vi "Modify Users.vi"(8 "error In":errorcluster) -> (0 "error Out":errorcluster)   [LabVIEW 2018]
uses:
  Control/Control 7.ctl
panel:
  in  "Login":bool
  in  "New User Type":enum16{"VVDN TECH", "Operator", "QA"}(ring)
  out "Current User Type":enum16{"VVDN TECH", "Operator", "QA"}(ring)
  in  "Stop Button":bool
  in  "Enum":T1
  in  "Selection":string(combo)
  out "Login":bool
  in  "Password":string
  in  "User Name":string(combo)="VVDN TECH"
  in  "Project-Name":string="LensTuning"
  in  "Modify User":bool
  # "MODIFY USERS"
  # "Modify User Details"
  # "Admin Login"
  # "Select User to Modify"
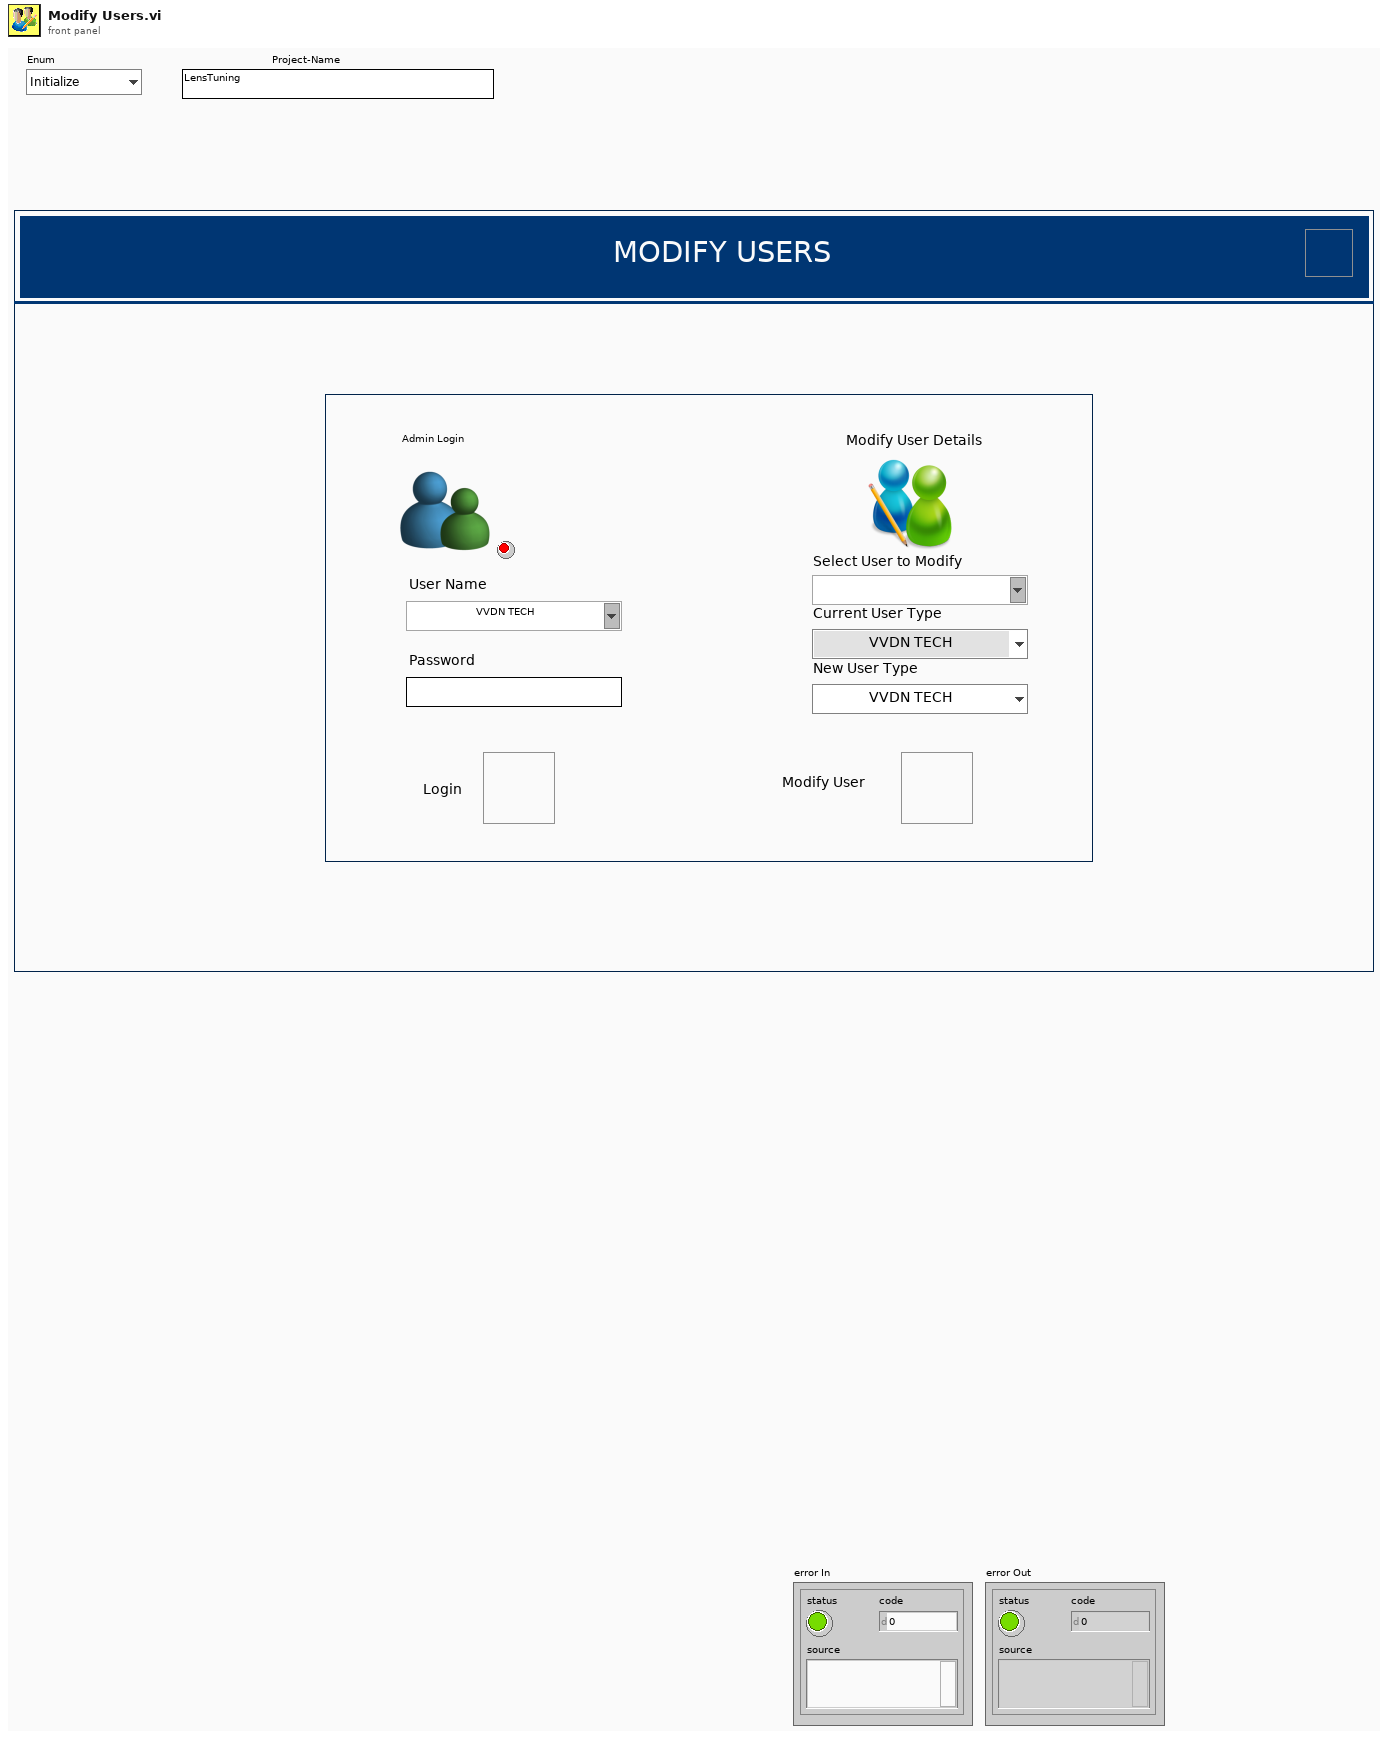
[diagram p1: front panel]
types:
  T1 = typedef "Control 7.ctl" = enum16{"Initialize", "Poll", "Login", "Add User", "Exit"}
  T2 = cluster{"Default User ":string, "Default Password":string, "Default User Type":u16}[]
  T3 = cluster{"Default User ":string, "Default Password":string, "Default User Type":u16}
  T4 = enum32{"Invalid", "Standard", "Closed", "Hidden", "Minimized", "Maximized"}
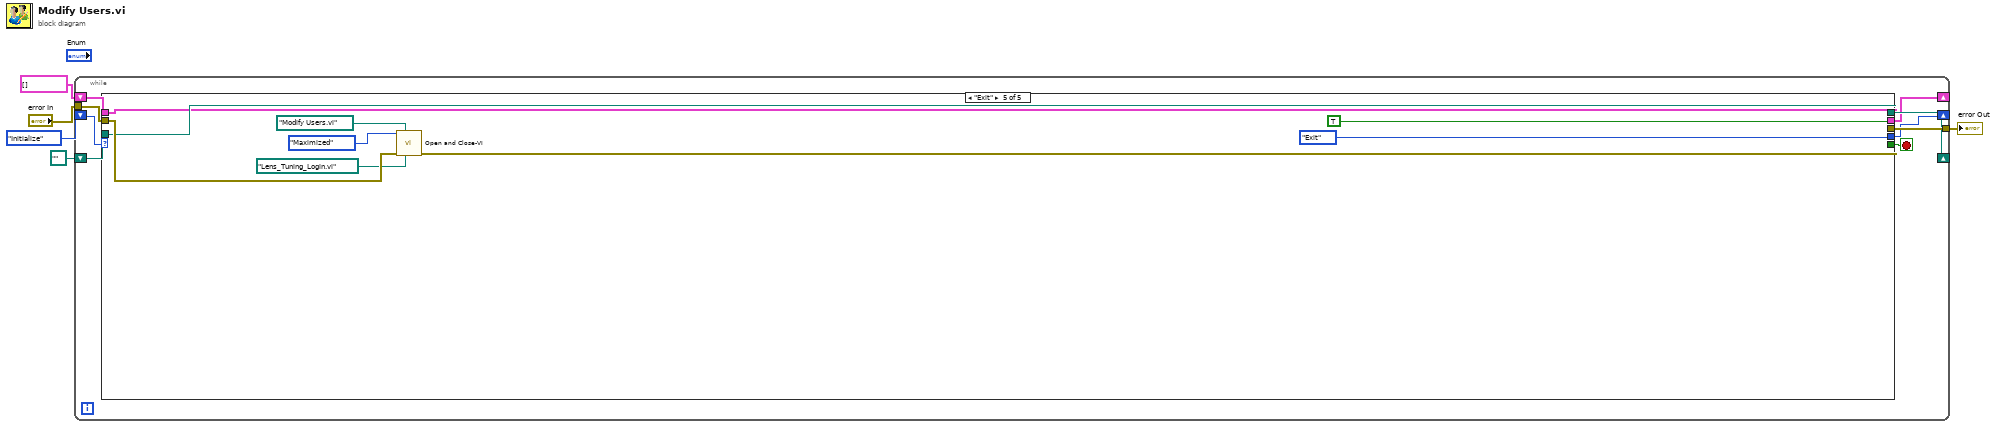
[diagram p0: block diagram]
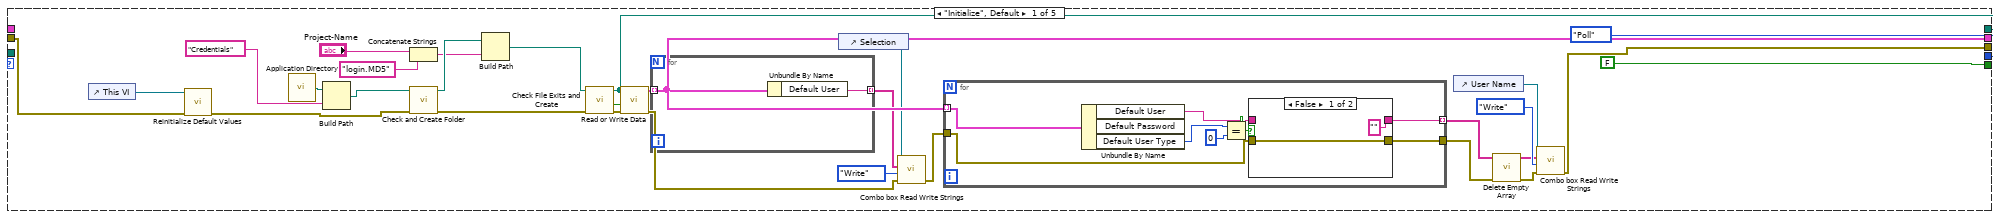
[diagram p2: hidden frame]
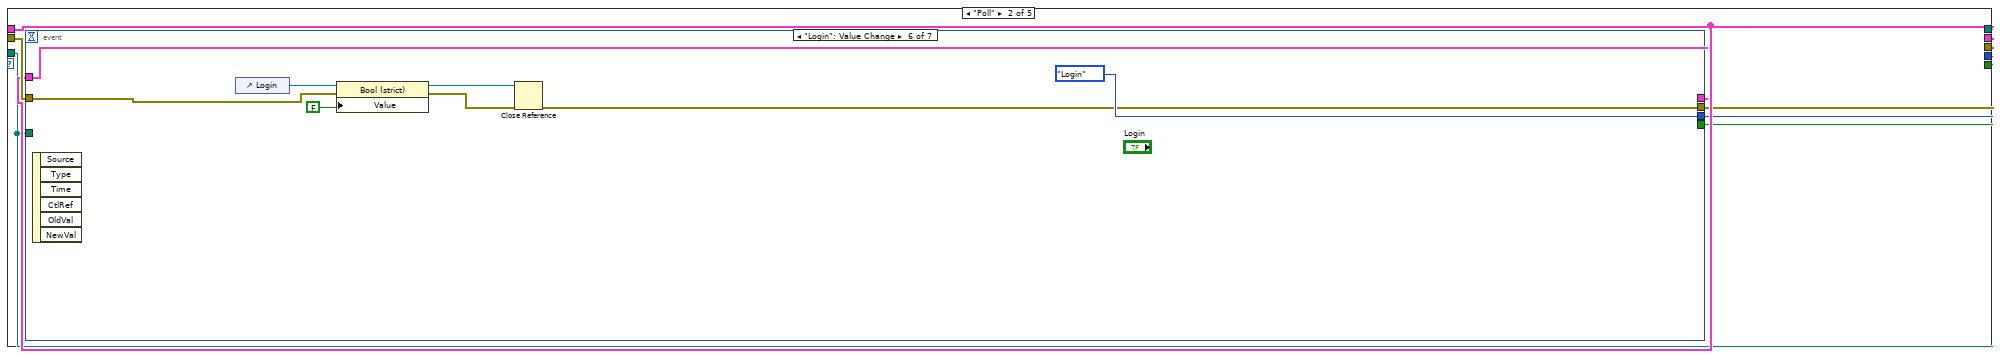
[diagram p4: hidden frame]
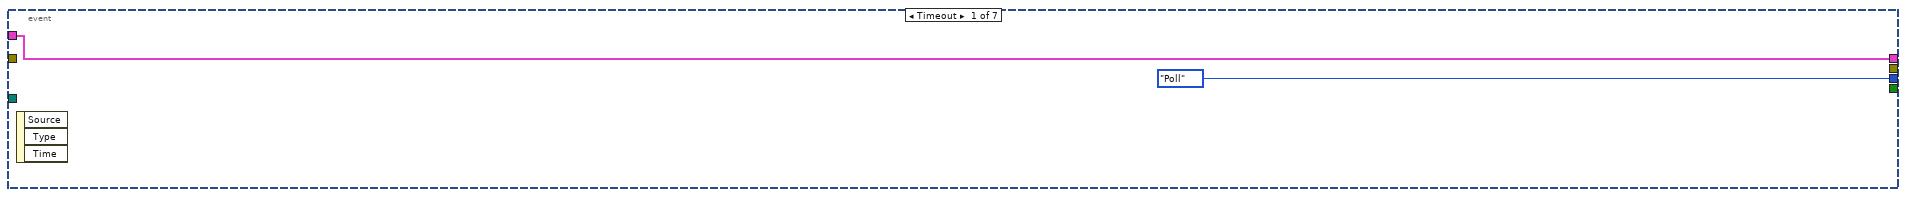
[diagram p5: hidden frame]
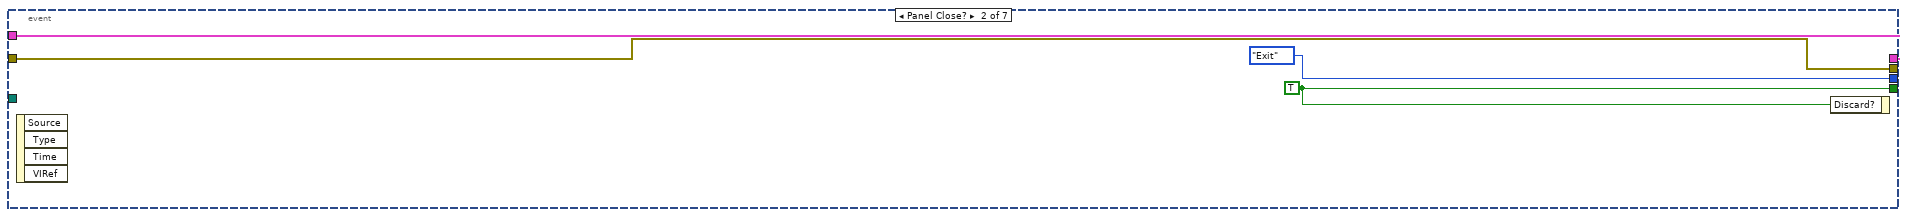
[diagram p6: hidden frame]
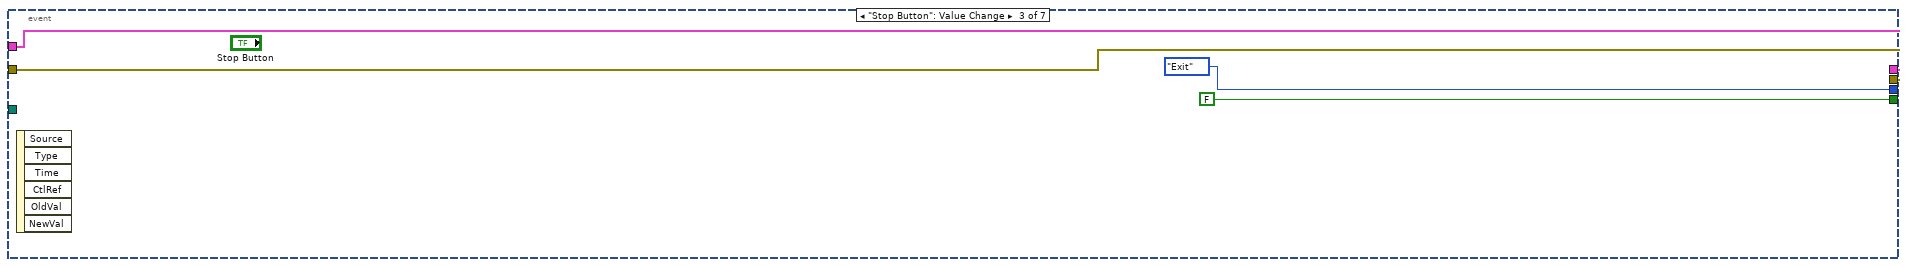
[diagram p7: hidden frame]
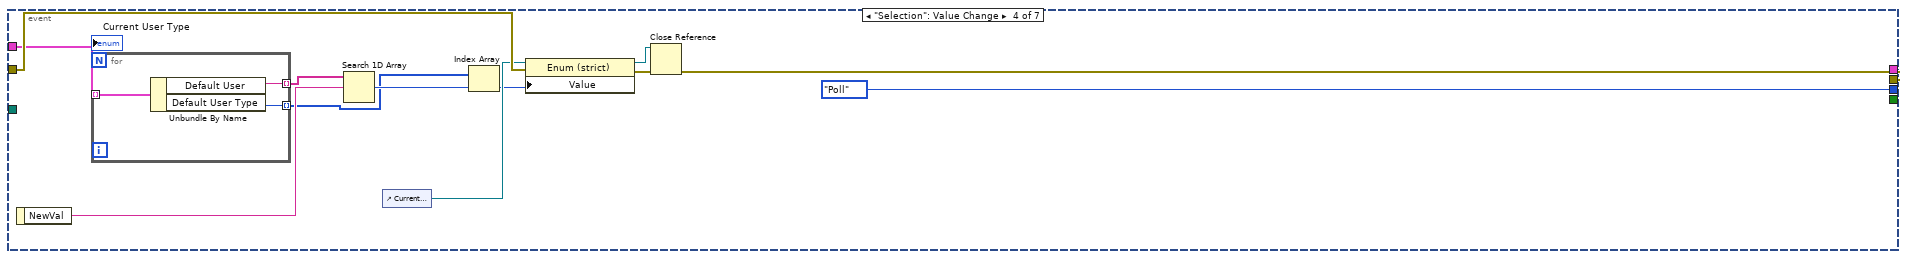
[diagram p8: hidden frame]
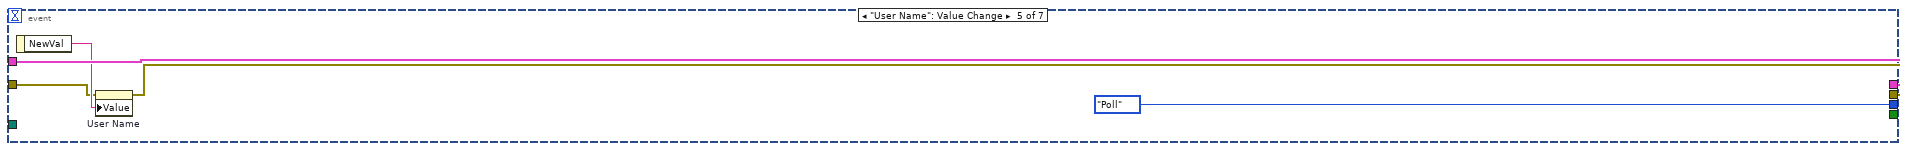
[diagram p9: hidden frame]
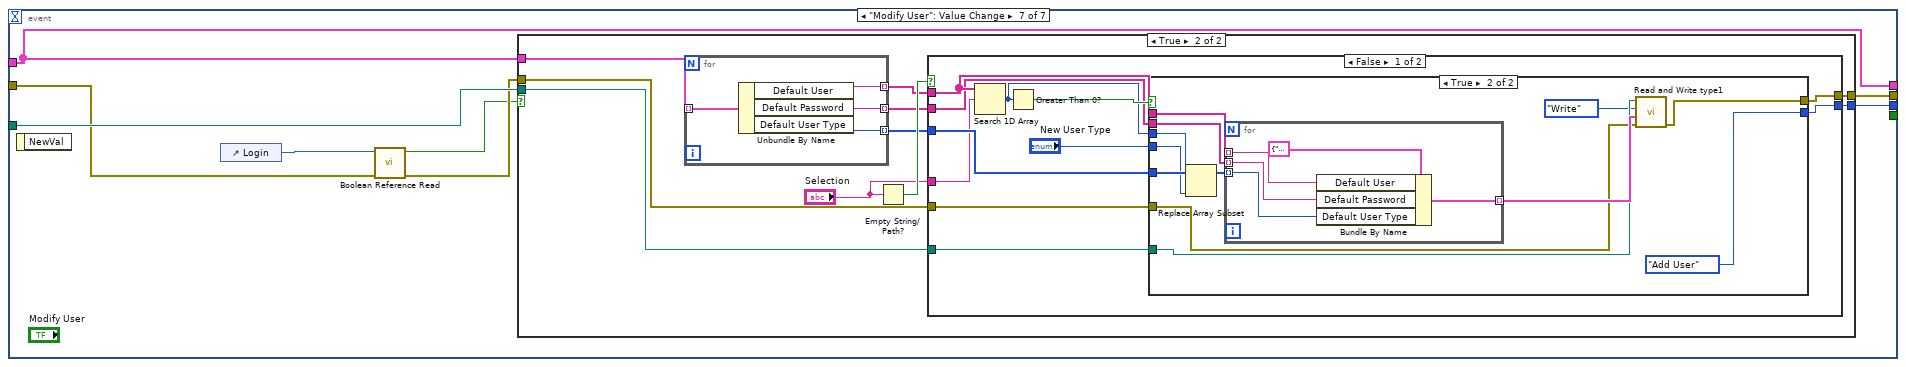
[diagram p10: hidden frame]
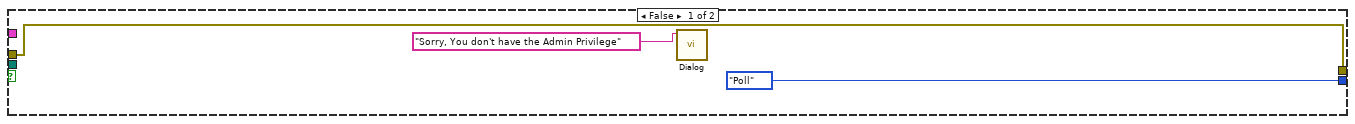
[diagram p11: hidden frame]
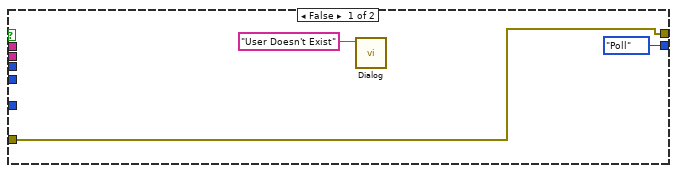
[diagram p12: hidden frame]
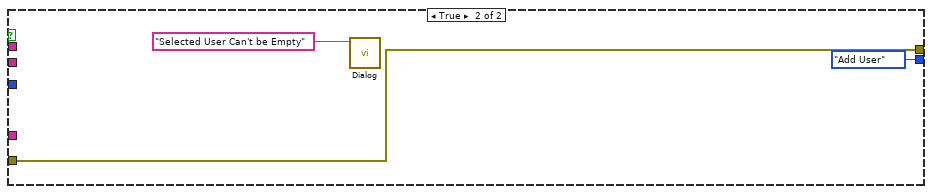
[diagram p13: hidden frame]
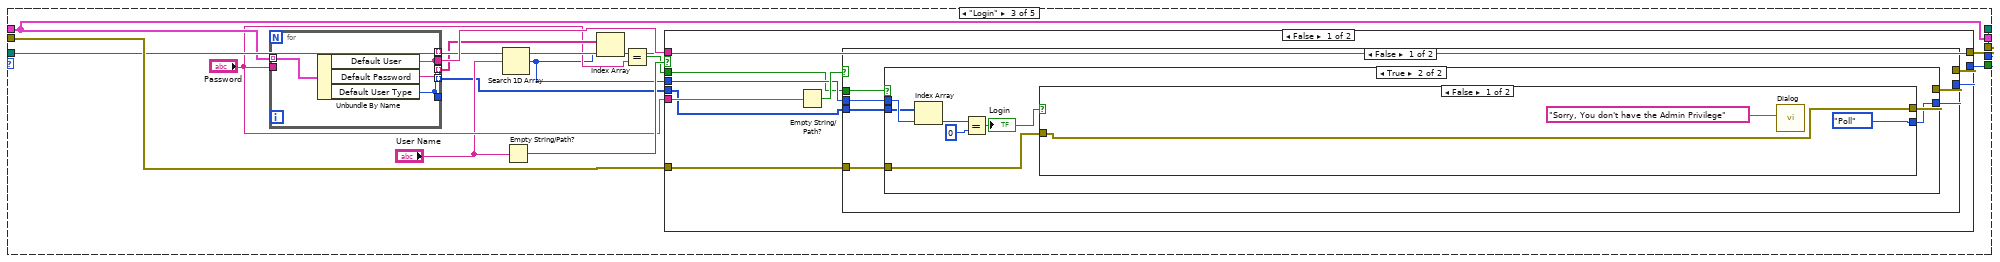
[diagram p14: hidden frame]
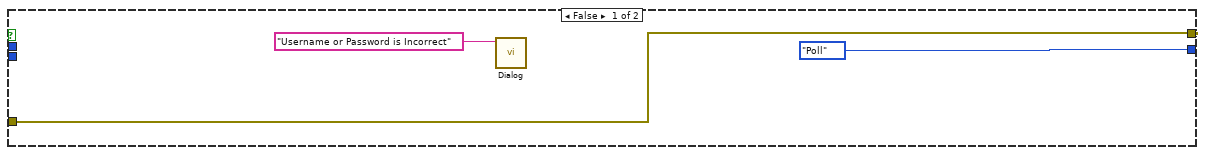
[diagram p15: hidden frame]
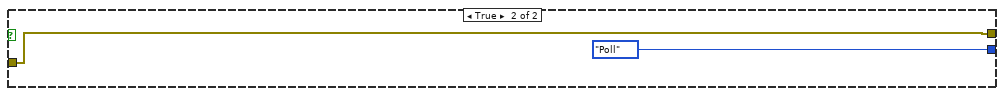
[diagram p16: hidden frame]
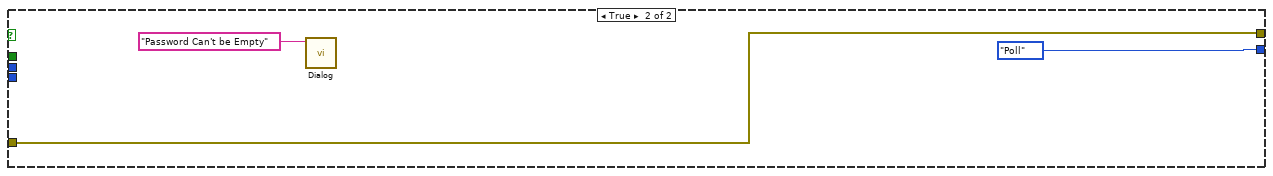
[diagram p17: hidden frame]
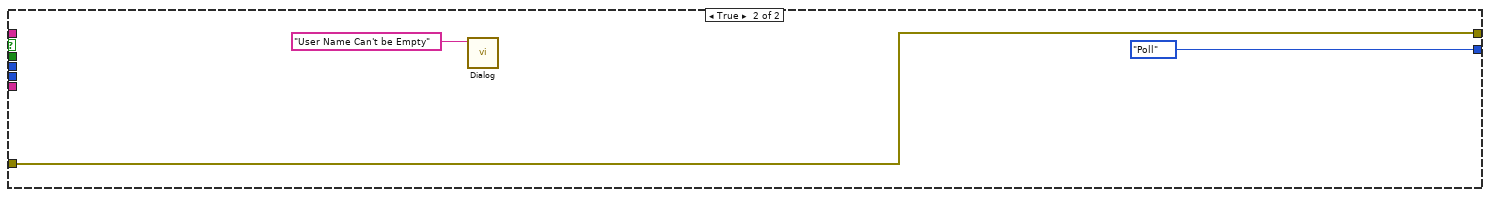
[diagram p18: hidden frame]
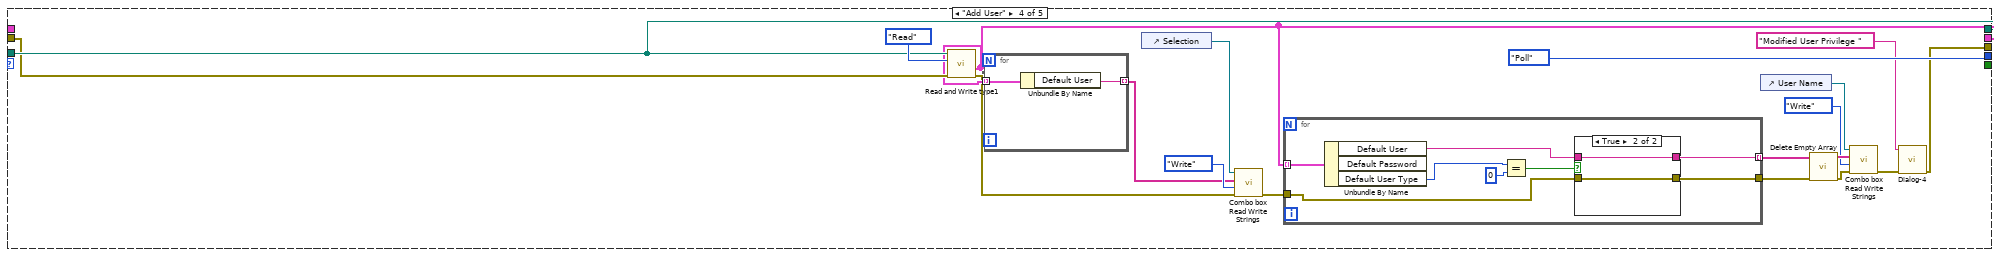
[diagram p19: hidden frame]
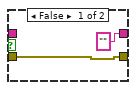
[diagram p20: hidden frame]
diagram:
  n1 = while {
    shift-right: [w10] -> _
    shift-left: Control_7."Initialize" ("Enum") -> [w14]
    tunnel: "error In" -> [w13]
    tunnel: [w12] -> w4
    shift-right: [w6] -> _
    shift-left: T2 [] ("User Details") -> [w11]
    shift-right: [w8] -> _
    shift-left: path "" ("Path Out") -> [w7]
    stop <- w9 stop-if-true
    n2 = case shown="\"Exit\"" w14 {
      tunnel: w13 -> [w26 w64 w176 w232 w257]
      tunnel: [w16 w62 w173 w228 w256] -> w12
      tunnel: w11 -> [_ w63 w170 _ w250]
      tunnel: [Control_7."Poll" ("Enum") w61 w174 Control_7."Poll" ("Enum") Control_7."Exit" ("Enum")] -> w10
      tunnel: [FALSE ("Discard?") w60 _ _ TRUE ("Discard?")] -> w9
      tunnel: [w31 w59 w171 w233 w251] -> w8
      tunnel: w7 -> [_ w59 w171 w233 w251]
      tunnel: [w28 w63 w170 w229 w250] -> w6
      frame "Initialize", Default {
        n3 = control-ref of="This VI"() -> (w27:refnum<vi>)
        n4 = call "Reinitialize Default Values.vi"("error in (no error)"=w26, "VI in"=w27) -> ("error out"=w25:errorcluster)  [unwired: 9 in]
        n5 = call <vilib>:"Application Directory.vi"() -> ("Application Directory"=w42:path)
        n6 = Build Path(base path=w42, name or relative path="Credentials") -> (appended path=w38:path)
        n7 = Concatenate Strings("Project-Name", "login.MD5" ("string")) -> (w36:string)
        n8 = call "Check and Create Folder.vi"("error in (no error)"=w25, "Path In"=w38) -> ("error out"=w35:errorcluster, "Path Out"=w37:path)  [unwired: 7 in, 1 out]
        n9 = Build Path(base path=w37, name or relative path=w36) -> (appended path=w34:path)
        n10 = call "Check File Exits and Create.vi"("error in"=w35, "Path In"=w34) -> ("error out"=w43:errorcluster, "file exists?"=w44:bool, "Path Out"=w31:path)  [unwired: 6 in, 1 out]
        n11 = call "Read or Write Data.vi"("error in"=w43, "file exists?"=w44, "Path Out"=w31) -> ("error out"=w23:errorcluster, "User Details"=w28:T2)  [unwired: 7 in]
        n12 = for {
          tunnel: w28 -> [w58] mode=indexing
          tunnel: [w57] -> w21 mode=indexing
          n13 = Unbundle By Name(w58) -> ("Default User"=w57:string)
        }
        n14 = control-ref of="Selection"() -> (w20:refnum<vi>)
        n15 = call "Combo box Read Write Strings.vi"("error in (no error)"=w23, "Enum"=enum16{"Read", "Write"}."Write", "Strings []"=w21, "ComboBox in"=w20) -> ("error out"=w22:errorcluster)  [unwired: 6 in, 1 out]
        n16 = for {
          tunnel: w28 -> [w52] mode=indexing
          tunnel: w22 -> [w47]
          tunnel: [w46] -> w30 mode=indexing
          tunnel: [w45] -> w29
          n17 = Unbundle By Name(w52) -> ("Default User"=w48:string, "Default User Type"=w51:u16)  [unwired: 1 out]
          n18 = Equal?(x=w51, y=u16 0) -> (x = y?=w49:bool)
          n19 = case shown="False" w49 {
            tunnel: w48 -> [_ w56]
            tunnel: ["" ("Default User") w56] -> w46
            tunnel: [w53 w55] -> w45
            tunnel: w47 -> [w53 w55]
            frame False {
            }
            frame True {
            }
          }
        }
        n20 = control-ref of="User Name"() -> (w19:refnum<vi>)
        n21 = call "Delete Empty Array.vi"("error in"=w29, "Array in"=w30) -> ("error out"=w17:errorcluster, "Array out"=w15:string[])  [unwired: 8 in]
        n22 = call "Combo box Read Write Strings.vi"("error in (no error)"=w17, "Enum"=enum16{"Read", "Write"}."Write", "Strings []"=w15, "ComboBox in"=w19) -> ("error out"=w16:errorcluster)  [unwired: 6 in, 1 out]
      }
      frame "Poll" {
        n23 = event shown="[5] \"Login\": Value Change" {
          selector: _ -> [_ _ _ _ _ _ _]
          dyn-events: _ -> [_ _ _ _ _ _ _]
          timeout: _ -> [_ _ _ _ _ _ _]
          tunnel: w64 -> [_ w70 w72 w86 w91 w98 w105]
          tunnel: w63 -> [w65 w69 w74 w80 w94 w102 w109]
          tunnel: [w65 w69 w74 _ w94 w102 w109] -> _
          tunnel: [_ w70 w72 w83 w90 w95 w108] -> w62
          tunnel: [Control_7."Poll" ("Enum") Control_7."Exit" ("Enum") Control_7."Exit" ("Enum") Control_7."Poll" ("Enum") Control_7."Poll" ("Enum") Control_7."Login" ("Enum") w110] -> w61
          tunnel: [_ w68 FALSE ("Discard?") _ _ _ _] -> w60
          tunnel: w59 -> [_ _ _ _ _ _ w107]
          event Timeout {
            n24 = event-data() -> ()  [unwired: 1 in, 3 out]
          }
          event Panel Close? {
            w68 = TRUE ("Discard?")
            n25 = event-data() -> ()  [unwired: 1 in, 4 out]
            n26 = event-data("Discard?"=w68) -> ()  [unwired: 1 in, 1 out]
          }
          event "Stop Button": Value Change {
            n27 = event-data() -> ()  [unwired: 1 in, 6 out]
          }
          event "Selection": Value Change {
            n28 = event-data() -> ("NewVal"=w78:string)  [unwired: 1 in]
            n29 = for {
              tunnel: w80 -> [w89] mode=indexing
              tunnel: [w88] -> w79 mode=indexing
              tunnel: [w87] -> w76 mode=indexing
              n30 = Unbundle By Name(w89) -> ("Default User"=w88:string, "Default User Type"=w87:u16)
            }
            n31 = Search 1D Array(1D array=w79, element=w78) -> (index of element=w77:i32)  [unwired: 1 in]
            n32 = control-ref of="Current User Type"() -> (w81:refnum<vi>)
            n33 = Index Array(array=w76, index=w77) -> (element=w75:u16)
            n34 = property class="Enum (strict)"(reference=w81, error in=w86, "Value"=w75) -> (reference out=w85:refnum<vi>, error out=w84:errorcluster)
            n35 = Close Reference(reference=w85, error in (no error)=w84) -> (error out=w83:errorcluster)
          }
          event "User Name": Value Change {
            n36 = event-data() -> ("NewVal"=w92:string)  [unwired: 1 in]
            n37 = property on="User Name" class="CmbBox"(error in=w91, "Value"=w92) -> (error out=w90:errorcluster)  [unwired: 1 in, 1 out]
          }
          event "Login": Value Change {
            n38 = event-data() -> ()  [unwired: 1 in, 6 out]
            n39 = control-ref of="Login"() -> (w100:refnum<vi>)
            n40 = property class="Bool (strict)"(reference=w100, error in=w98, "Value"=FALSE) -> (reference out=w96:refnum<vi>, error out=w97:errorcluster)
            n41 = Close Reference(reference=w96, error in (no error)=w97) -> (error out=w95:errorcluster)
          }
          event "Modify User": Value Change {
            n42 = event-data() -> ()  [unwired: 1 in, 1 out]
            n43 = control-ref of="Login"() -> (w106:refnum<vi>)
            n44 = call "Boolean Reference Read.vi"("error in (no error)"=w105, "Boolean in"=w106) -> ("error out"=w104:errorcluster, "Value"=w103:bool)  [unwired: 8 in]
            n45 = case shown="True" w103 {
              tunnel: [Control_7."Poll" ("Enum") w122] -> w110
              tunnel: w109 -> [_ w116]
              tunnel: w104 -> [w112 w120]
              tunnel: [w112 w119] -> w108
              tunnel: w107 -> [_ w115]
              frame False {
                n46 = call "Dialog.vi"("Status"="Sorry, You don't have the Admin Privilege") -> ()  [unwired: 10 in, 1 out]
              }
              frame True {
                n47 = for {
                  tunnel: w116 -> [w127] mode=indexing
                  tunnel: [w126] -> w121 mode=indexing
                  tunnel: [w125] -> w118 mode=indexing
                  tunnel: [w124] -> w117 mode=indexing
                  n48 = Unbundle By Name(w127) -> ("Default User"=w126:string, "Default Password"=w125:string, "Default User Type"=w124:u16)
                }
                n49 = Empty String/Path?(string/path="Selection") -> (empty?=w123:bool)
                n50 = case shown="False" w123 {
                  tunnel: [w137 Control_7."Add User" ("Enum")] -> w122
                  tunnel: w121 -> [w134 _]
                  tunnel: w120 -> [w136 w159]
                  tunnel: [w135 w159] -> w119
                  tunnel: w118 -> [w132 _]
                  tunnel: w117 -> [w131 _]
                  tunnel: w115 -> [w130 _]
                  tunnel: "Selection" -> [w129 _]
                  frame False {
                    n51 = Search 1D Array(1D array=w134, element=w129) -> (index of element=w133:i32)  [unwired: 1 in]
                    n52 = Greater Than 0?(x=w133) -> (x > 0?=w138:bool)
                    n53 = case shown="True" w138 {
                      tunnel: [Control_7."Poll" ("Enum") Control_7."Add User" ("Enum")] -> w137
                      tunnel: w136 -> [w141 w149]
                      tunnel: [w141 w148] -> w135
                      tunnel: w134 -> [_ w147]
                      tunnel: w133 -> [_ w144]
                      tunnel: w132 -> [_ w146]
                      tunnel: w131 -> [_ w145]
                      tunnel: w130 -> [_ w151]
                      tunnel: "New User Type" -> [_ w143]
                      frame False {
                        n54 = call "Dialog.vi"("Status"="User Doesn't Exist") -> ()  [unwired: 10 in, 1 out]
                      }
                      frame True {
                        n55 = Replace Array Subset(array=w145, new element=w143, index=w144) -> (w142:u16[])
                        n56 = for {
                          tunnel: [w157] -> w152 mode=indexing
                          tunnel: w147 -> [w156] mode=indexing
                          tunnel: w146 -> [w155] mode=indexing
                          tunnel: w142 -> [w154] mode=indexing
                          n57 = Bundle By Name(cluster=T3 {"Default User "="", "Default Password"="", "Default User Type"=0}, "Default User"=w156, "Default Password"=w155, "Default User Type"=w154) -> (w157:T3)
                        }
                        n58 = call "Read and Write type1.vi"("error in"=w149, "IN"=w152, "Enum"=enum16{"Init", "Read", "Write"}."Write", "Path Out"=w151) -> ("error out"=w148:errorcluster)  [unwired: 6 in, 1 out]
                      }
                    }
                  }
                  frame True {
                    n59 = call "Dialog.vi"("Status"="Selected User Can't be Empty") -> ()  [unwired: 10 in, 1 out]
                  }
                }
              }
            }
          }
        }
      }
      frame "Login" {
        n60 = for {
          tunnel: w170 -> [w180] mode=indexing
          tunnel: [w179] -> w172
          tunnel: "Password" -> [_]
          tunnel: [w177] -> _
          tunnel: [w179] -> w169 mode=indexing
          tunnel: [w178] -> w168 mode=indexing
          tunnel: [w177] -> w163 mode=indexing
          n61 = Unbundle By Name(w180) -> ("Default User"=w179:string, "Default Password"=w178:string, "Default User Type"=w177:u16)
        }
        n62 = Search 1D Array(1D array=w169, element="User Name") -> (index of element=w162:i32)  [unwired: 1 in]
        n63 = Empty String/Path?(string/path="User Name") -> (empty?=w175:bool)
        n64 = Index Array(array=w168, index=w162) -> (element=w167:string)
        n65 = Equal?(x=w167, y="Password") -> (x = y?=w165:bool)
        n66 = case shown="False" w175 {
          tunnel: w176 -> [w186 w214]
          tunnel: [w184 Control_7."Poll" ("Enum")] -> w174
          tunnel: [w185 w214] -> w173
          tunnel: w172 -> [_ _]
          tunnel: "Password" -> [w188 _]
          tunnel: w162 -> [w183 _]
          tunnel: w165 -> [w182 _]
          tunnel: w163 -> [w181 _]
          frame False {
            n67 = Empty String/Path?(string/path=w188) -> (empty?=w187:bool)
            n68 = case shown="False" w187 {
              tunnel: w186 -> [w194 w213]
              tunnel: [w193 w213] -> w185
              tunnel: [w192 Control_7."Poll" ("Enum")] -> w184
              tunnel: w183 -> [w191 _]
              tunnel: w182 -> [w190 _]
              tunnel: w181 -> [w189 _]
              frame False {
                n69 = case shown="True" w190 {
                  tunnel: w194 -> [w196 w204]
                  tunnel: [w196 w203] -> w193
                  tunnel: [Control_7."Poll" ("Enum") w202] -> w192
                  tunnel: w191 -> [_ w200]
                  tunnel: w189 -> [_ w199]
                  frame False {
                    n70 = call "Dialog.vi"("Status"="Username or Password is Incorrect") -> ()  [unwired: 10 in, 1 out]
                  }
                  frame True {
                    n71 = Index Array(array=w199, index=w200) -> (element=w198:u16)
                    n72 = Equal?(x=w198, y=u16 0) -> (x = y?=w201:bool)
                    "Login" <- w201
                    n73 = case shown="False" w201 {
                      tunnel: w204 -> [w207 w210]
                      tunnel: [w207 w210] -> w203
                      tunnel: [Control_7."Poll" ("Enum") Control_7."Poll" ("Enum")] -> w202
                      frame False {
                        n74 = call "Dialog.vi"("Status"="Sorry, You don't have the Admin Privilege") -> ()  [unwired: 10 in, 1 out]
                      }
                      frame True {
                      }
                    }
                  }
                }
              }
              frame True {
                n75 = call "Dialog.vi"("Status"="Password Can't be Empty") -> ()  [unwired: 10 in, 1 out]
              }
            }
          }
          frame True {
            n76 = call "Dialog.vi"("Status"="User Name Can't be Empty") -> ()  [unwired: 10 in, 1 out]
          }
        }
      }
      frame "Add User" {
        n77 = call "Read and Write type1.vi"("error in"=w232, "Enum"=enum16{"Init", "Read", "Write"}."Read", "Path Out"=w233) -> ("error out"=w226:errorcluster, "OUT"=w229:T2)  [unwired: 7 in]
        n78 = for {
          tunnel: w229 -> [w249] mode=indexing
          tunnel: [w248] -> w222 mode=indexing
          n79 = Unbundle By Name(w249) -> ("Default User"=w248:string)
        }
        n80 = control-ref of="Selection"() -> (w224:refnum<vi>)
        n81 = call "Combo box Read Write Strings.vi"("error in (no error)"=w226, "Enum"=enum16{"Read", "Write"}."Write", "Strings []"=w222, "ComboBox in"=w224) -> ("error out"=w225:errorcluster)  [unwired: 6 in, 1 out]
        n82 = for {
          tunnel: w229 -> [w243] mode=indexing
          tunnel: w225 -> [w238]
          tunnel: [w237] -> w231 mode=indexing
          tunnel: [w236] -> w230
          n83 = Unbundle By Name(w243) -> ("Default User"=w239:string, "Default User Type"=w242:u16)  [unwired: 1 out]
          n84 = Equal?(x=w242, y=u16 0) -> (x = y?=w240:bool)
          n85 = case shown="True" w240 {
            tunnel: w239 -> [_ w247]
            tunnel: ["" ("Default User") w247] -> w237
            tunnel: [w244 w246] -> w236
            tunnel: w238 -> [w244 w246]
            frame False {
            }
            frame True {
            }
          }
        }
        n86 = control-ref of="User Name"() -> (w218:refnum<vi>)
        n87 = call "Delete Empty Array.vi"("error in"=w230, "Array in"=w231) -> ("error out"=w221:errorcluster, "Array out"=w219:string[])  [unwired: 8 in]
        n88 = call "Combo box Read Write Strings.vi"("error in (no error)"=w221, "Enum"=enum16{"Read", "Write"}."Write", "Strings []"=w219, "ComboBox in"=w218) -> ("error out"=w220:errorcluster)  [unwired: 6 in, 1 out]
        n89 = call "Dialog-4.vi"("error in"=w220, "Status"="Modified User Privilege ") -> ("error out"=w228:errorcluster)  [unwired: 8 in, 1 out]
      }
      frame "Exit" {
        n90 = call "Open and Close-VI.vi"("State"=T4."Maximized", "Close VI"=path "Modify Users.vi", "error in"=w257, "Open VI"=path "Lens_Tuning_Login.vi") -> ("error out"=w256:errorcluster)  [unwired: 11 in]
      }
    }
  }
  "error Out" <- w4
